vi "Set Path.vi"(10 "Path":path, 11 "Sender in":refnum<class "Sender.lvclass">) -> (3 "Sender out":refnum<class "Sender.lvclass">)   [LabVIEW 2021, in "jettl.lvlib" / "Sender.lvlib" / "Sender.lvclass"]
uses:
  Sender.lvclass
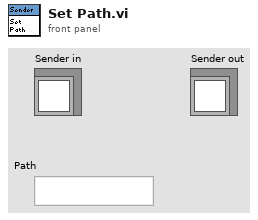
[diagram p1: front panel]
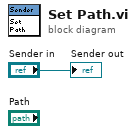
[diagram p0: block diagram]
diagram:
  "Sender out" <- "Sender in"
